vi "rtout_getTriggerConfig.vi"(0 "connection ID":i32, 1 "axis":i32, 5 "error in":errorcluster) -> (12 "polarity":i32, 14 "connection ID":i32, 15 "axis_out":i32, 16 "higher":i32, 17 "lower":i32, 18 "epsilon":i32, 19 "error out":errorcluster)   [LabVIEW 2016]
doc: "Get the real time output trigger config"
panel:
  out "params_cluster":cluster{"axis":i32}
  in  "Params_cluster":cluster{"integer":i32}
  in  "results_cluster":T1
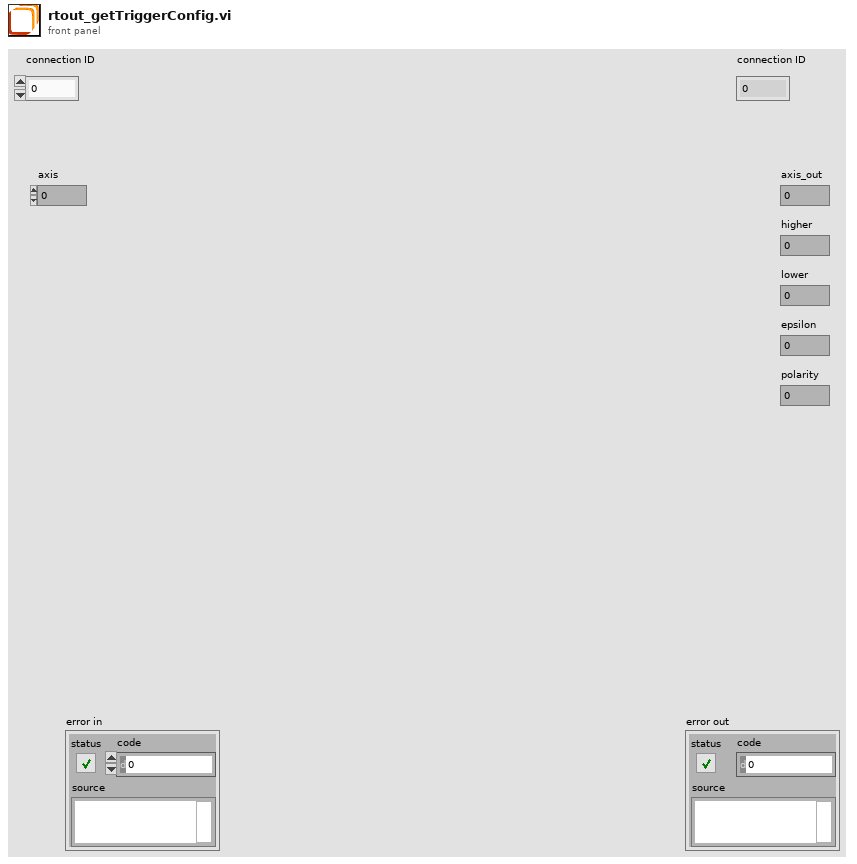
[diagram p1: front panel]
types:
  T1 = cluster{"errNo":i32, "higher":i32, "lower":i32, "epsilon":i32, "polarity":i32}
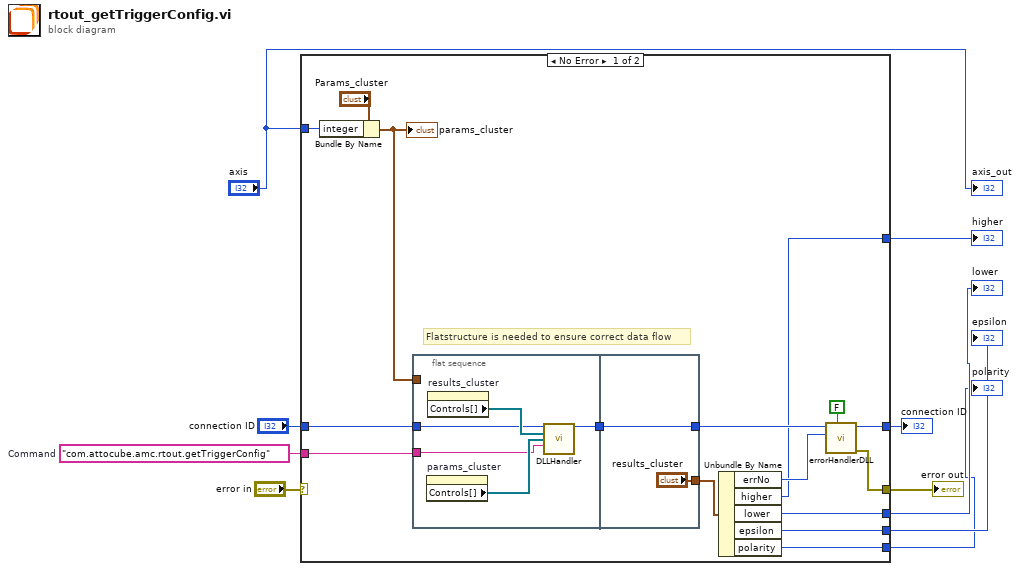
[diagram p0: block diagram]
diagram:
  w8 = "com.attocube.amc.rtout.getTriggerConfig"  # Command
  n1 = case shown="No Error" "error in" {
    selector: "error in" -> [_ w35]
    tunnel: [w25 w35] -> w10
    tunnel: w8 -> [w20 _]
    tunnel: [w19 w34] -> w7
    tunnel: "connection ID" -> [w18 w34]
    tunnel: "axis" -> [w15 _]
    tunnel: [w14 _] -> w4
    tunnel: [w13 _] -> w3
    tunnel: [w12 _] -> w2
    tunnel: [w11 _] -> w1
    frame No Error {
      # "Flatstructure is needed to ensure correct data flow"
      n2 = Bundle By Name(cluster="Params_cluster", "integer"=w15) -> (w16:cluster{"integer":i32})
      "params_cluster" <- w16
      n3 = flat-sequence {
        tunnel: [w31] -> w22
        tunnel: w20 -> [w28]
        tunnel: w18 -> [w27]
        tunnel: w16 -> [_]
        tunnel: ["results_cluster"] -> w23
        tunnel: [w33] -> w24
        tunnel: w22 -> [w33]
        frame #0 {
          n4 = property on="params_cluster" class="Clust (strict)"() -> ("Controls[]"=w29:refnum<vi>[])  [unwired: 2 in, 2 out]
          n5 = property on="results_cluster" class="Clust (strict)"() -> ("Controls[]"=w30:refnum<vi>[])  [unwired: 2 in, 2 out]
          n6 = call "DLLHandler.vi"("connection ID"=w27, "results_cluster"=w30, "params_cluster"=w29, "method"=w28) -> ("connection ID out"=w31:i32)  [unwired: 10 in, 1 out]
        }
        frame #1 {
        }
      }
      n7 = Unbundle By Name(w23) -> ("errNo"=w17:i32, "higher"=w14:i32, "lower"=w13:i32, "epsilon"=w12:i32, "polarity"=w11:i32)
      n8 = call "errorHandlerDLL.vi"("show popup"=FALSE, "error number"=w17, "connection ID"=w24) -> ("error out"=w25:errorcluster, "connection ID"=w19:i32)  [unwired: 7 in]
    }
    frame Error {
    }
  }
  "error out" <- w10
  "connection ID" <- w7
  "higher" <- w4
  "lower" <- w3
  "epsilon" <- w2
  "polarity" <- w1
  "axis_out" <- "axis"
